vi "getFitting.vi"(8 "error in (no error)":errorcluster, 11 "LaguerreDeconEngineClass in":refnum<class "LaguerreDeconEngineClass.lvclass">) -> (0 "error out":errorcluster, 2 "Fitting":dbl[](array[numeric]), 3 "LaguerreDeconEngineClass out":refnum<class "LaguerreDeconEngineClass.lvclass">)   [LabVIEW 2020, in "LaguerreDeconEngineClass.lvclass"]
uses:
  LaguerreDeconEngineClass.lvclass
  LaguerreDeconEngineClass.lvclass/LaguerreDeconEngineClass.ctl
  <vilib>/Analysis/2dsp.llb/1D Convolution (DBL).vi
  <vilib>/Analysis/NI_AALPro.lvlib
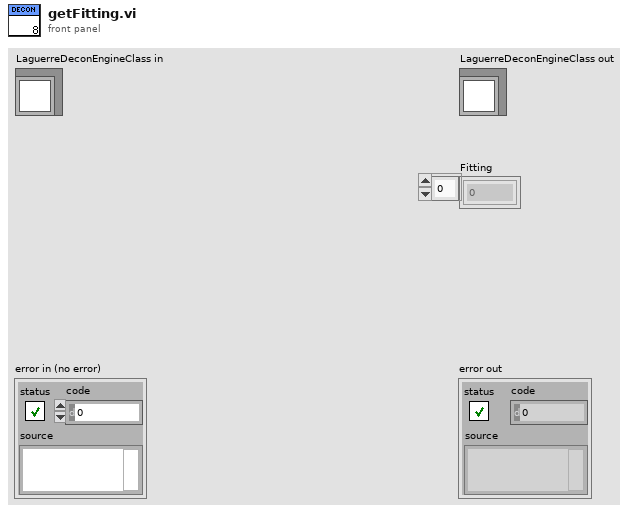
[diagram p1: front panel]
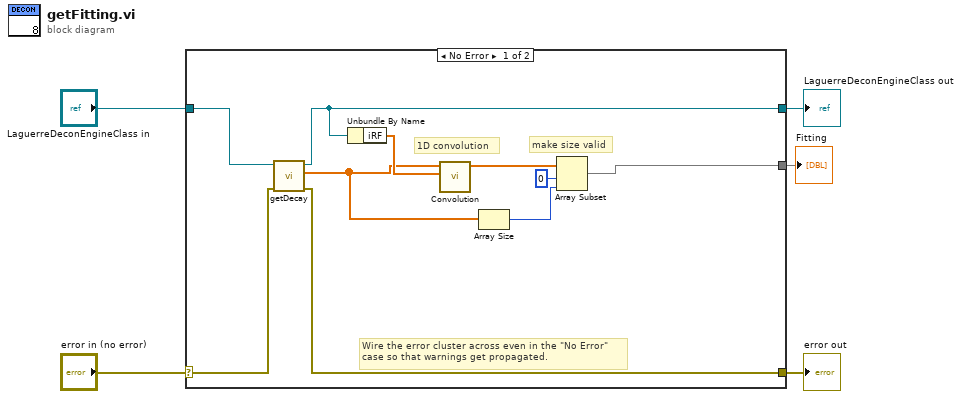
[diagram p0: block diagram]
diagram:
  n1 = case shown="No Error" "error in (no error)" {
    selector: "error in (no error)" -> [w15 w17]
    tunnel: [w14 w17] -> w4
    tunnel: [w12 w16] -> w2
    tunnel: "LaguerreDeconEngineClass in" -> [w13 w16]
    tunnel: [w9 _] -> w1
    frame No Error {
      # "make size valid"
      # "1D convolution"
      # "Wire the error cluster across even in the \"No Error\"\ncase so that warnings get propagated."
      n2 = call "getDecay.vi"("error in (no error)"=w15, "LaguerreDeconClass in"=w13) -> ("error out"=w14:errorcluster, "Decay"=w7:dbl[], "LaguerreDeconClass out"=w12:refnum<class "LaguerreDeconEngineClass.lvclass">)  [unwired: 7 in]
      n3 = Unbundle By Name(w12) -> ("iRF"=w11:dbl[])
      n4 = call-poly <vilib>:"Convolution.vi"("Y"=w11, "X"=w7) -> ("X * Y"=w10:dbl[])  [unwired: 8 in, 1 out]
      n5 = Array Size(array=w7) -> (size(s)=w6:i32)
      n6 = Array Subset(array=w10, index=0, length=w6) -> (w9:dbl[])
    }
    frame Error {
    }
  }
  "error out" <- w4
  "LaguerreDeconEngineClass out" <- w2
  "Fitting" <- w1
